vi "Pre Launch Init.vi"(11 "Logger in":refnum<class "Logger.lvclass">) -> (0 "error out":errorcluster, 3 "Logger out":refnum<class "Logger.lvclass">)   [LabVIEW 2017, in "Logger.lvlib" / "Logger.lvclass"]
doc: "(<B>Filename</B>: Actor Framework.lvlib:Actor.lvclass:Pre Launch Init.vi)\n\nDefines behavior that occurs after the Launch Nested Actor method is invoked but before the actor's Actor Core method begins running.\n\nBy default, this method does nothing. A descendant class may override it to define behavior."
uses:
  Logger.lvclass
  C:/Program Files (x86)/National Instruments/LabVIEW 2017/vi.lib/ActorFramework/Actor/Actor.lvclass
  <vilib>/ActorFramework/Actor/Actor.lvclass/Actor.ctl
  <vilib>/ActorFramework/Message Enqueuer/Message Enqueuer.lvclass/Message Enqueuer.ctl
  Logger.lvclass/Logger.ctl
  config/Logger Configuration.lvclass/Logger Configuration.ctl
  config/Read Logging Settings.vi
  <vilib>/ActorFramework/Message Enqueuer/Init from Existing Queue.vi
  <vilib>/ActorFramework/Message Enqueuer/Enqueue.vi
  Logger Messages/Configure AMQP Client Msg/Configure AMQP Client Msg.lvclass
  C:/Program Files (x86)/National Instruments/LabVIEW 2017/vi.lib/ActorFramework/Message/Message.lvclass
  Logger Messages/Create New File Msg/Create New File Msg.lvclass
  <vilib>/ActorFramework/Message Priority Queue/Priority Enqueue.vi
  <vilib>/ActorFramework/Actor/Actor.lvclass
  <vilib>/ActorFramework/Message Enqueuer/Message Enqueuer.lvclass
  config/Logger Configuration.lvclass
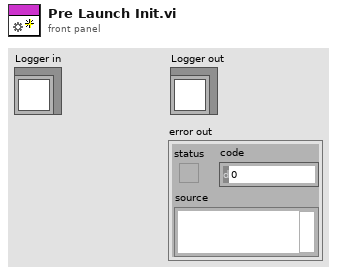
[diagram p1: front panel]
types:
  T1 = cluster{"File Name":string, "Upload Files to SystemLink Server":bool, "Max Samples Per File":i32, "Folder Location":path, "Logging":bool}
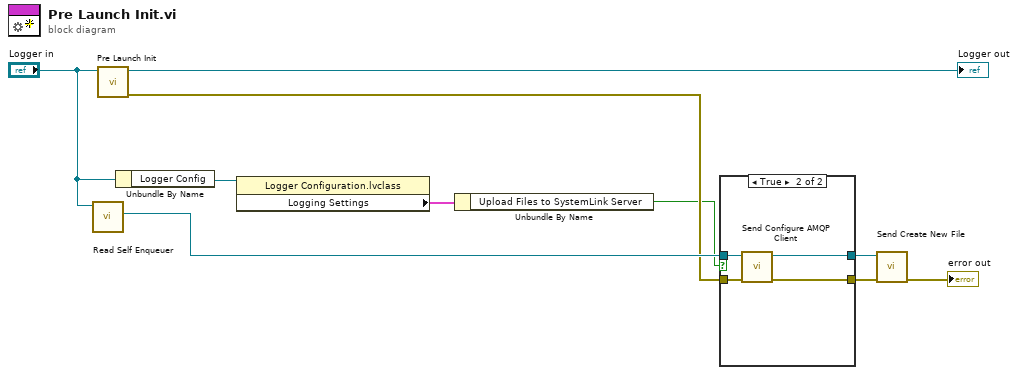
[diagram p0: block diagram]
diagram:
  n1 = call <vilib>:"Read Self Enqueuer.vi"("Actor"="Logger in") -> ("Self Enqueuer"=w8:refnum<class "Message Enqueuer.lvclass">)  [unwired: 10 in]
  n2 = call-parent "Pre Launch Init.vi"("Actor in"="Logger in") -> ("error out"=w7:errorcluster, "Actor out"=→"Logger out":refnum<class "Logger.lvclass">)  [unwired: 9 in]
  n3 = Unbundle By Name("Logger in") -> ("Logger Config"=w3:refnum<class "Logger Configuration.lvclass">)
  n4 = property class="Logger Configuration.lvclass"(reference=w3) -> ("Logging Settings"=w2:T1)  [unwired: 1 in, 2 out]
  n5 = Unbundle By Name(w2) -> ("Upload Files to SystemLink Server"=w1:bool)
  n6 = case shown="True" w1 {
    tunnel: [w12 w16] -> w9
    tunnel: w8 -> [w12 w15]
    tunnel: w7 -> [w11 w14]
    tunnel: [w11 w13] -> w6
    frame False {
    }
    frame True {
      n7 = call "Send Configure AMQP Client.vi"("error in (no error)"=w14, "Message Enqueuer"=w15) -> ("error out"=w13:errorcluster, "Message Enqueuer out"=w16:refnum<class "Message Enqueuer.lvclass">)  [unwired: 8 in]
    }
  }
  n8 = call "Send Create New File.vi"("error in (no error)"=w6, "Message Enqueuer"=w9) -> ("error out"=→"error out":errorcluster)  [unwired: 8 in, 1 out]
